vi "update.name.request.vi"(8 "error in":errorcluster, 11 "Title":string) -> (0 "error out":errorcluster, 1 "Request":string)   [LabVIEW 2020, in "Run.lvclass"]
uses:
  Run.lvclass
  Run.lvclass/Run.ctl
  94201847-ea5e-4d83-86fc-2cdbeb98d53f.vi
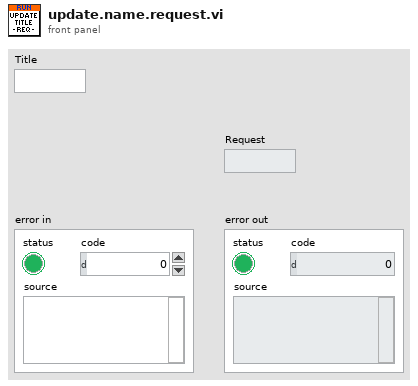
[diagram p1: front panel]
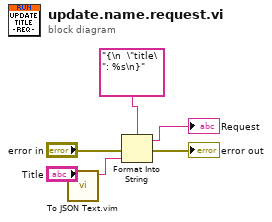
[diagram p0: block diagram]
diagram:
  n1 = call "To JSON Text.vim"("Anything"="Title") -> ("<JSON>"=w1:string)  [unwired: 9 in, 1 out]
  n2 = Format Into String(format string="{\n  \"title\": %s\n}", error in="error in", w1) -> (resulting string=→"Request":string, error out=→"error out":errorcluster)  [unwired: 1 in]
